vi "Write SerialData.vi"(8 "error in (no error)":errorcluster, 10 "SerialData":refnum<class "Data.lvclass">[](array[class]), 11 "PAS Data in":refnum<class "PAS Data.lvclass">) -> (0 "error out":errorcluster, 3 "PAS Data out":refnum<class "PAS Data.lvclass">)   [LabVIEW 2014]
uses:
  PAS Data.lvclass
  Data/Data.lvclass
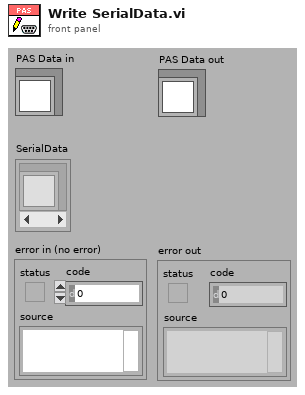
[diagram p1: front panel]
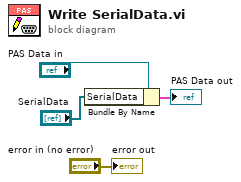
[diagram p0: block diagram]
diagram:
  n1 = Bundle By Name(cluster="PAS Data in", "SerialData"="SerialData") -> (→"PAS Data out":cluster{})
  "error out" <- "error in (no error)"
